vi "Get_AcquisitionData.vi"(8 "error in (no error)":errorcluster, 9 "Variant":variant, 11 "Avantes in":refnum<class "Avantes.lvclass">) -> (0 "error out":errorcluster, 2 "Data":T1(array[cluster]), 3 "Avantes out":refnum<class "Avantes.lvclass">, 5 "Time":dbl[](array[numeric]))   [LabVIEW 2018, in "Avantes.lvclass"]
uses:
  <instrlib>/Classes/CCD/Avantes/Avantes.lvclass
panel:
  out "a_pTimeLabel":u32
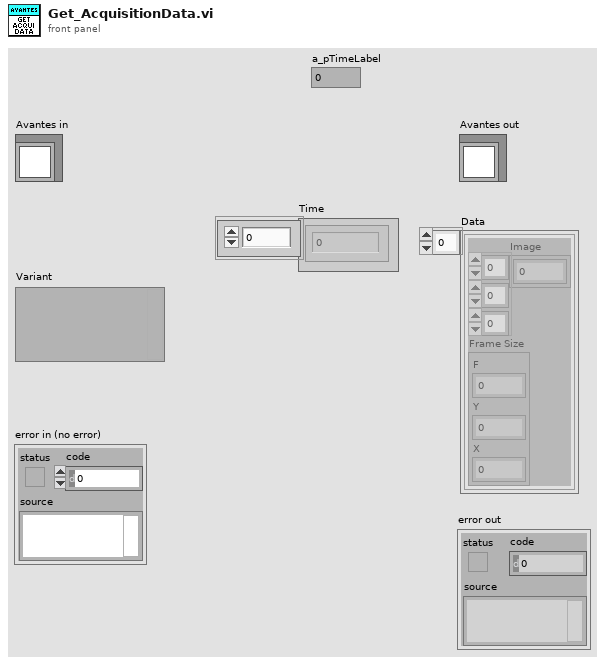
[diagram p1: front panel]
types:
  T1 = cluster{"Image":dbl[][][], "Frame Size":cluster{"F":i32, "Y":i32, "X":i32}}[]
  T2 = cluster{"Image":dbl[][][], "Frame Size":cluster{"F":i32, "Y":i32, "X":i32}}
  T3 = cluster{"Frames":i32, "Start Pixel":u16, "Stop Pixel":u16}
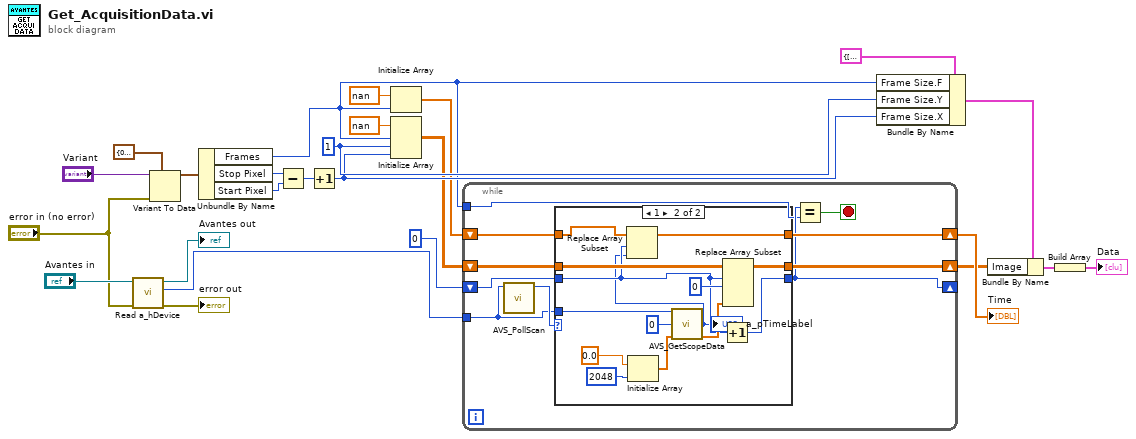
[diagram p0: block diagram]
diagram:
  w14 = 1 ("dimension size")
  n1 = call-dynamic "Read a_hDevice.vi"("error in (no error)"="error in (no error)", "Avantes in"="Avantes in") -> ("error out"=→"error out":errorcluster, "a_hDevice"=w10:i32, "Avantes out"=→"Avantes out":refnum<class "Avantes.lvclass">)  [unwired: 7 in]
  n2 = Variant To Data(error in="error in (no error)", type=T3 {"Frames"=0, "Start Pixel"=0, "Stop Pixel"=0}, Variant="Variant") -> (data=w22:T3)  [unwired: 1 out]
  n3 = Unbundle By Name(w22) -> ("Frames"=w8:i32, "Stop Pixel"=w17:u16, "Start Pixel"=w16:u16)
  n4 = Subtract(x=w17, y=w16) -> (x-y=w18:u16)
  n5 = Increment(x=w18) -> (x+1=w13:u16)
  n6 = Initialize Array(nan ("element"), w8) -> (w7:dbl[])
  n7 = Initialize Array(nan ("element"), w8, w14, w13) -> (w11:dbl[][][])
  n8 = while {
    shift-right: [w33] -> w6
    shift-left: w7 -> [w34]
    shift-right: [w31] -> w3
    shift-left: w11 -> [w32]
    shift-right: [w28] -> _
    shift-left: 0 ("Frames") -> [w30]
    tunnel: w10 -> [w27]
    tunnel: w8 -> [w26]
    stop <- w29 stop-if-true
    n9 = call <instrlib>:"AVS_PollScan.vi"("a_hDevice"=w27) -> ("Output Value"=w35:i32)  [unwired: 8 in]
    n10 = case shown="1" w35 {
      tunnel: w34 -> [w38 w51]
      tunnel: [w38 w50] -> w33
      tunnel: w32 -> [w36 w49]
      tunnel: [w36 w47] -> w31
      tunnel: w30 -> [w37 w41]
      tunnel: [w37 w46] -> w28
      tunnel: w27 -> [_ w40]
      frame 0, Default {
      }
      frame 1 {
        n11 = Initialize Array(0.0 ("element"), 2048 ("dimension size")) -> (w45:dbl[])
        n12 = call <instrlib>:"AVS_GetScopeData.vi"("a_hDevice"=w40, "a_pTimeLabel"=u32 0, "a_pSpectrum"=w45) -> ("a_pTimeLabel"=w39:u32, "a_pSpectrum"=w42:dbl[])  [unwired: 10 in, 1 out]
        "a_pTimeLabel" <- w39
        n13 = Replace Array Subset(array=w51, new element=w39, index=w41) -> (w50:dbl[])
        n14 = Increment(x=w41) -> (x+1=w46:i32)
        n15 = Replace Array Subset(array=w49, new element=w42, index (dim 0)=w41, index (dim 1)=0 ("disabled index (row)")) -> (w47:dbl[][][])  [unwired: 1 in]
      }
    }
    n16 = Equal?(x=w28, y=w26) -> (x = y?=w29:bool)
  }
  "Time" <- w6
  n17 = Bundle By Name(cluster=T2 {"Image"=[], "Frame Size"={"F"=0, "Y"=0, "X"=0}} ("Cluster"), "Frame Size.F"=w8, "Frame Size.Y"=w14, "Frame Size.X"=w13) -> (w4:T2)
  n18 = Bundle By Name(cluster=w4, "Image"=w3) -> (w2:T2)
  n19 = Build Array(w2) -> (→"Data":T1)
